vi "CreateRotationX.vi"(8 "error in (no error)":errorcluster, 9 "radians":dbl, 11 "3D Scene in":refnum<class "3D Scene.lvclass">) -> (0 "error out":errorcluster, 2 "modelview rotated":T1, 3 "3D Scene out":refnum<class "3D Scene.lvclass">)   [LabVIEW 2015, in "3D Scene.lvclass"]
uses:
  3D Scene.lvclass
  <vilib>/Analysis/Matrix/Datatypes/RealMatrix.ctl
  <vilib>/Analysis/Matrix/NI_Matrix.lvlib
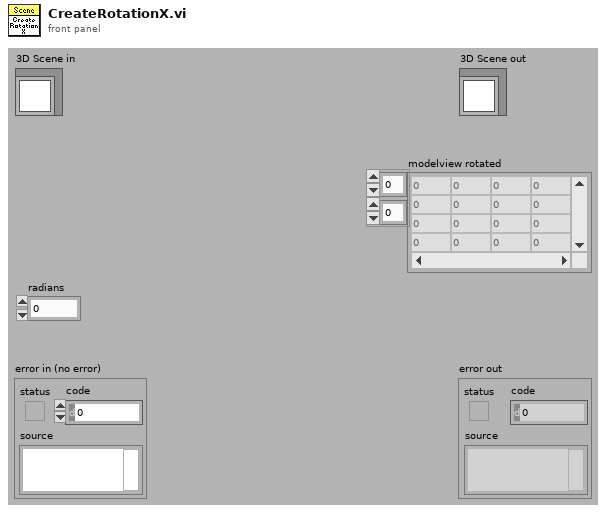
[diagram p1: front panel]
types:
  T1 = typedef "NI_Matrix.lvlib/RealMatrix.ctl" = dbl[][]
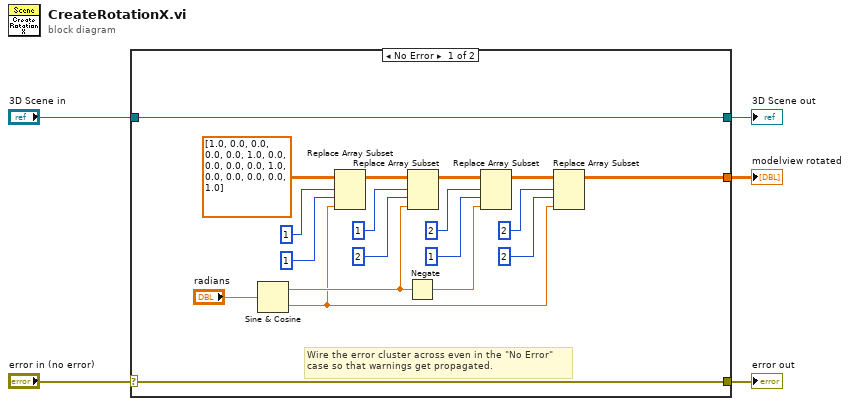
[diagram p0: block diagram]
diagram:
  n1 = case shown="No Error" "error in (no error)" {
    selector: "error in (no error)" -> [w23 w26]
    tunnel: [w23 w26] -> w4
    tunnel: [w24 w25] -> w2
    tunnel: "3D Scene in" -> [w24 w25]
    tunnel: [w7 _] -> w1
    frame No Error {
      # "Wire the error cluster across even in the \"No Error\"\ncase so that warnings get propagated."
      n2 = Sine & Cosine(0:"radians") -> (1:w11:dbl, 2:w9:dbl)
      n3 = Replace Array Subset(array=T1 [[1.0, 0.0, 0.0, 0.0], [0.0, 1.0, 0.0, 0.0], [0.0, 0.0, 1.0, 0.0], [0.0, 0.0, 0.0, 1.0]] ("A"), new element=w9, index (row)=1, index (col)=1 ("disabled index (col)")) -> (w22:T1)
      n4 = Negate(x=w11) -> (-x=w10:dbl)
      n5 = Replace Array Subset(array=w22, new element=w11, index (row)=1 ("disabled index (row)"), index (col)=2 ("disabled index (col)")) -> (w21:T1)
      n6 = Replace Array Subset(array=w21, new element=w10, index (row)=2, index (col)=1 ("disabled index (col)")) -> (w20:T1)
      n7 = Replace Array Subset(array=w20, new element=w9, index (row)=2, index (col)=2 ("disabled index (col)")) -> (w7:T1)
    }
    frame Error {
    }
  }
  "error out" <- w4
  "3D Scene out" <- w2
  "modelview rotated" <- w1
